vi "נא בחר ממסר.vi"(0 "Enable":bool=TRUE, 5 "error in (no error)":errorcluster) -> (12 "בחר הכל":bool, 14 "P - N/L":bool, 15 "G - H/J":bool, 16 "D - E/F":bool, 17 "A - B/C":bool, 18 "OK":bool, 19 "error out":errorcluster)   [LabVIEW 2014]
doc: "Displays a standard dialog box that prompts users to enter information, such as a user name and password.\n--------------------\n\nThis Express VI is configured as follows:\n\nMessage to Display to the User:נא בחר ממסר לבדוק\nThe inputs are: \nCheckbox: A - B/C\nCheckbox: D - E/F\nCheckbox: G - H/J\nCheckbox: P - N/L"
panel:
  in  "בחר הכל":bool
  in  "P - N/L":bool
  in  "G - H/J":bool
  in  "D - E/F":bool
  in  "A - B/C":bool
  out "String":string="נא בחר ממסר לבדוק"
  in  "Cancel":bool
  in  "OK2":bool
  in  "OK1":bool
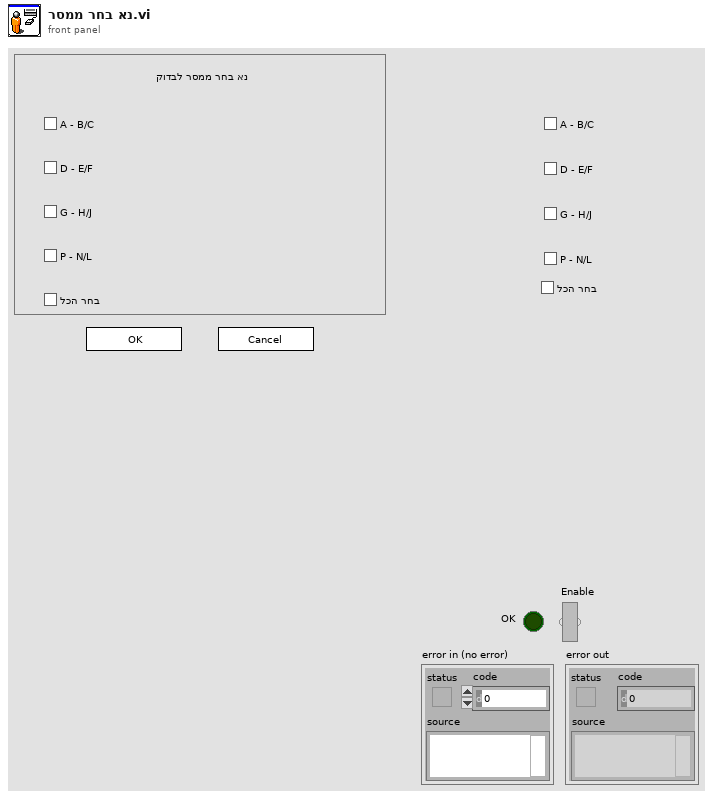
[diagram p1: front panel]
types:
  T1 = cluster{"Input Name":string, "Input Data Type":i32}[]
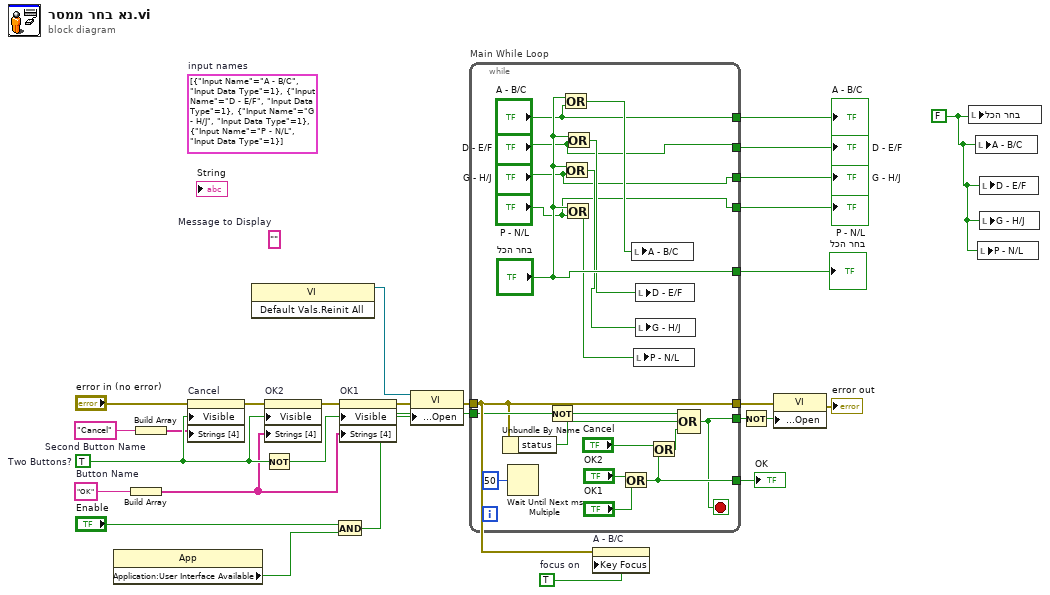
[diagram p0: block diagram]
diagram:
  w1 = FALSE
  w7 = TRUE  # focus on
  (unwired) T1 [{"Input Name"="A - B/C", "Input Data Type"=1}, {"Input Name"="D - E/F", "Input Data Type"=1}, {"Input Name"="G - H/J", "Input Data Type"=1}, {"Input Name"="P - N/L", "Input Data Type"=1}]  # input names
  w19 = "Cancel"  # Second Button Name
  w17 = "OK"  # Button Name
  (unwired) ""  # Message to Display
  w27 = TRUE  # Two Buttons?
  n1 = property class="App"() -> ("Application:User Interface Available"=w9:bool)  [unwired: 2 in, 2 out]
  n2 = Build Array(w17) -> (w18:string[])
  n3 = Build Array(w19) -> (w20:string[])
  n4 = property on="Cancel" class="Bool"(error in="error in (no error)", "Visible"=w27, "Strings [4]"=w20) -> (error out=w24:errorcluster)  [unwired: 1 in, 1 out]
  n5 = invoke class="VI" method="Default Vals.Reinit All"() -> (reference out=w8:refnum<vi>)  [unwired: 3 in, 2 out]
  n6 = Not(x=w27) -> (.not. x?=w25:bool)
  n7 = property on="OK2" class="Bool"(error in=w24, "Visible"=w27, "Strings [4]"=w18) -> (error out=w23:errorcluster)  [unwired: 1 in, 1 out]
  n8 = And(x="Enable", y=w9) -> (x .and. y?=w10:bool)
  n9 = property on="OK1" class="Bool"(error in=w23, "Visible"=w25, "Strings [4]"=w18) -> (error out=w16:errorcluster)  [unwired: 1 in, 1 out]
  n10 = property class="VI"(reference=w8, error in=w16, "Front Panel Window:Open"=w10) -> (error out=w15:errorcluster)  [unwired: 1 out]
  n11 = while "Main While Loop" {
    tunnel: [w44] -> w26
    tunnel: w10 -> [w42]
    tunnel: [w40] -> w21
    tunnel: w15 -> [w39]
    tunnel: [w39] -> w13
    tunnel: ["A - B/C"] -> w6
    tunnel: ["D - E/F"] -> w5
    tunnel: ["G - H/J"] -> w2
    tunnel: ["P - N/L"] -> w4
    tunnel: ["בחר הכל"] -> w3
    stop <- w40 stop-if-true
    n12 = Unbundle By Name(w39) -> ("status"=w37:bool)
    n13 = Wait Until Next ms Multiple(millisecond multiple=u32 50) -> ()  [unwired: 1 out]
    n14 = Not(x=w42) -> (.not. x?=w41:bool)
    n15 = Or(x="בחר הכל", y="A - B/C") -> (x .or. y?=w35:bool)
    n16 = Or(x="בחר הכל", y="G - H/J") -> (x .or. y?=w33:bool)
    n17 = Or(x="בחר הכל", y="P - N/L") -> (x .or. y?=w32:bool)
    n18 = Or(x="בחר הכל", y="D - E/F") -> (x .or. y?=w34:bool)
    n19 = Or(x="OK2", y="OK1") -> (x .or. y?=w44:bool)
    n20 = local write "A - B/C"(w35) -> ()
    n21 = local write "P - N/L"(w32) -> ()
    n22 = local write "D - E/F"(w34) -> ()
    n23 = local write "G - H/J"(w33) -> ()
    n24 = Or(x="Cancel", y=w44) -> (x .or. y?=w38:bool)
    n25 = Compound Arithmetic op=OR(w41, w37, w38) -> (w40:bool)
  }
  "OK" <- w26
  "A - B/C" <- w6
  "D - E/F" <- w5
  "G - H/J" <- w2
  "P - N/L" <- w4
  "בחר הכל" <- w3
  n26 = property on="A - B/C" class="Bool (strict)"(error in=w15, "Key Focus"=w7) -> ()  [unwired: 1 in, 2 out]
  n27 = Not(x=w21) -> (.not. x?=w22:bool)
  n28 = property class="VI"(error in=w13, "Front Panel Window:Open"=w22) -> (error out=→"error out":errorcluster)  [unwired: 1 in, 1 out]
  n29 = local write "בחר הכל"(w1) -> ()
  n30 = local write "A - B/C"(w1) -> ()
  n31 = local write "P - N/L"(w1) -> ()
  n32 = local write "D - E/F"(w1) -> ()
  n33 = local write "G - H/J"(w1) -> ()
